vi "Set Actuator.vi"(8 "error in (no error)":errorcluster, 10 "Actuator":dbl) -> (0 "error out":errorcluster)   [LabVIEW 2021, in "Actuator Module.lvlib"]
doc: "_______\nCreated using Delacor User Event Scripter 1.0.0.6."
uses:
  Actuator Module.lvlib
  Set Actuator Argument--cluster.ctl
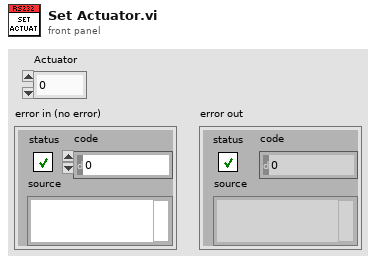
[diagram p1: front panel]
types:
  T1 = typedef "Actuator Module.lvlib/Set Actuator Argument--cluster.ctl" = cluster{"Actuator":dbl}
  T2 = typedef "Actuator Module.lvlib/Request Events--cluster.ctl" = cluster{"Stop":refnum<user-event>, "Set Actuator":refnum<user-event>}
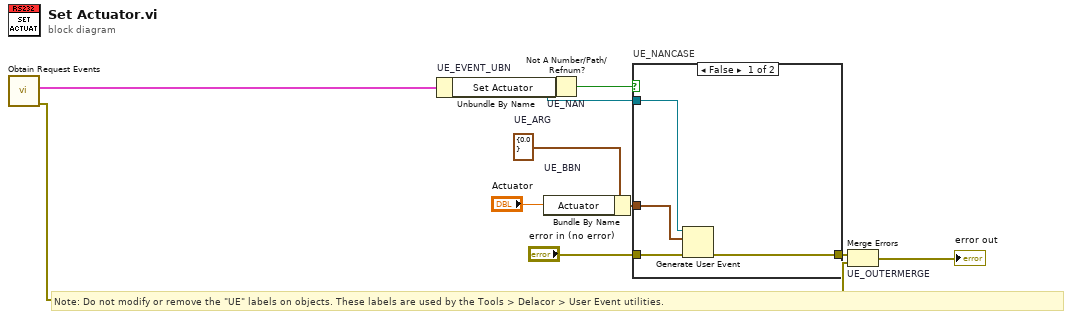
[diagram p0: block diagram]
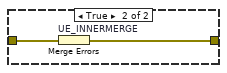
[diagram p2: hidden frame]
diagram:
  w4 = T1 {"Actuator"=0.0}  # UE_ARG
  # "Note: Do not modify or remove the \"UE\" labels on objects. These labels are used by the Tools > Delacor > User Event utilities."
  n1 = call "Obtain Request Events.vi"() -> ("error out"=w2:errorcluster, "Actuator Module Request Events"=w1:T2)  [unwired: 10 in]
  n2 = Unbundle By Name "UE_EVENT_UBN"(w1) -> ("Set Actuator"=w6:refnum<user-event>)
  n3 = Bundle By Name "UE_BBN"(cluster=w4, "Actuator"="Actuator") -> (w8:T1)
  n4 = Not A Number/Path/Refnum? "UE_NAN"(number/path/refnum=w6) -> (NaN/Path/Refnum?=w7:bool)
  n5 = case "UE_NANCASE" shown="False" w7 {
    tunnel: "error in (no error)" -> [w14 w16]
    tunnel: [w13 w15] -> w5
    tunnel: w6 -> [w12 _]
    tunnel: w8 -> [w11 _]
    frame False {
      n6 = Generate User Event(user event=w12, event data cluster=w11, error in=w14) -> (error out=w13:errorcluster)  [unwired: 1 in, 1 out]
    }
    frame True {
      n7 = Merge Errors "UE_INNERMERGE"(w16) -> (w15:errorcluster)
    }
  }
  n8 = Merge Errors "UE_OUTERMERGE"(w5, w2) -> (→"error out":errorcluster)
